vi "Lockin.Engine.vi"(8 "error in (no error)":errorcluster, 11 "Instrument.DAQ":refnum<class "Instrument.DAQ.lvclass">) -> (0 "error out":errorcluster, 1 "Downsampled Waveforms":T1, 2 "Results (X,Y,R,Theta,Mean)":T2 {"Results (Dictionary)"."value" format="%#_6p"}, 3 "Instrument.DAQ out":refnum<class "Instrument.DAQ.lvclass">, 5 "Continue DSP?":bool)   [LabVIEW 2019, in "Instrument.Lockin.lvlib" / "Instrument.DAQ.lvclass"]
uses:
  Instrument.DAQ.lvclass
  Typedefs/Results--Cluster.ctl
  Instrument.DAQ.lvclass/Instrument.DAQ.ctl
  DSP/DSP.lvclass
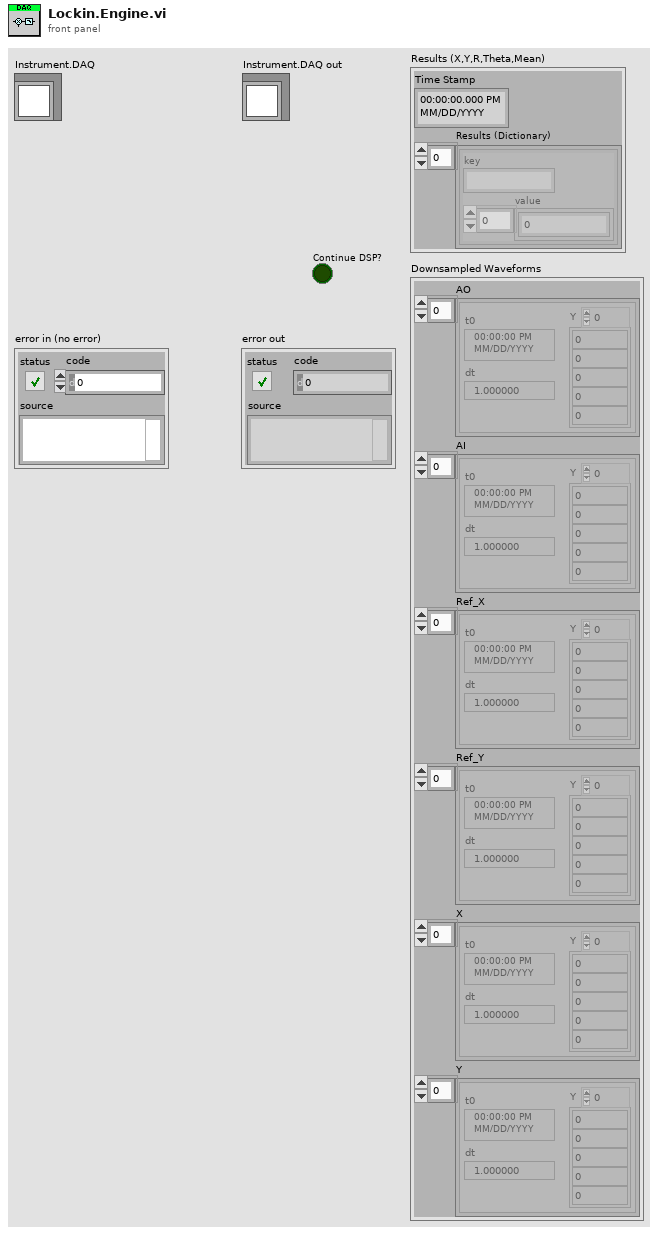
[diagram p1: front panel]
types:
  T1 = cluster{"AO":waveform(dbl)[], "AI":waveform(dbl)[], "Ref_X":waveform(dbl)[], "Ref_Y":waveform(dbl)[], "X":waveform(dbl)[], "Y":waveform(dbl)[]}
  T2 = typedef "Instrument.Lockin.lvlib/Instrument.DAQ.lvclass/Results--Cluster.ctl" = cluster{"Time Stamp":timestamp, "Results (Dictionary)":cluster{"key":string, "value":dbl[]}[]}
  T3 = typedef "Instrument.Lockin.lvlib/Instrument.DAQ.lvclass/PublicEvents--DAQ.getWaveforms.ctl" = cluster{"AO":waveform(dbl)[], "AI":waveform(dbl)[], "REF_X":waveform(dbl)[], "REF_Y":waveform(dbl)[], "X":waveform(dbl)[], "Y":waveform(dbl)[]}
  T4 = typedef "Instrument.Lockin.lvlib/Instrument.DAQ.lvclass/AI.Channel--Cluster--Array.ctl" = T5[]
  T5 = typedef "Instrument.Lockin.lvlib/Instrument.DAQ.lvclass/AI.Channel--Cluster.ctl" = cluster{"Enable?":bool, "Channel":i32, "References":u16[], "reference index":i32}
  T6 = typedef "Instrument.Lockin.lvlib/Instrument.DAQ.lvclass/REF.Channel--Cluster--Array.ctl" = T7[]
  T7 = typedef "Instrument.Lockin.lvlib/Instrument.DAQ.lvclass/REF.Channel--Cluster.ctl" = cluster{"Enable?":bool, "Channel":i32, "Frequency":dbl, "Phase":dbl, "TC":dbl, "Roll-Off":i32}
  T8 = typedef "Instrument.Lockin.lvlib/Instrument.DAQ.lvclass/DAQ.Sampling--Cluster.ctl" = cluster{"Sampling":T9, "Fs_Out":dbl}
  T9 = typedef "Instrument.Lockin.lvlib/Instrument.DAQ.lvclass/DAQ.Sampling.Sampling--Cluster.ctl" = cluster{"Fs":dbl, "#s":i32}
  T10 = typedef "DSP.lvclass/Results--Cluster.ctl" = cluster{"Time Stamp":timestamp, "Results (Dictionary)":T11[]}
  T11 = typedef "DSP.lvclass/Results Dictionary--Cluster.ctl" = cluster{"key":string, "value":dbl[]}
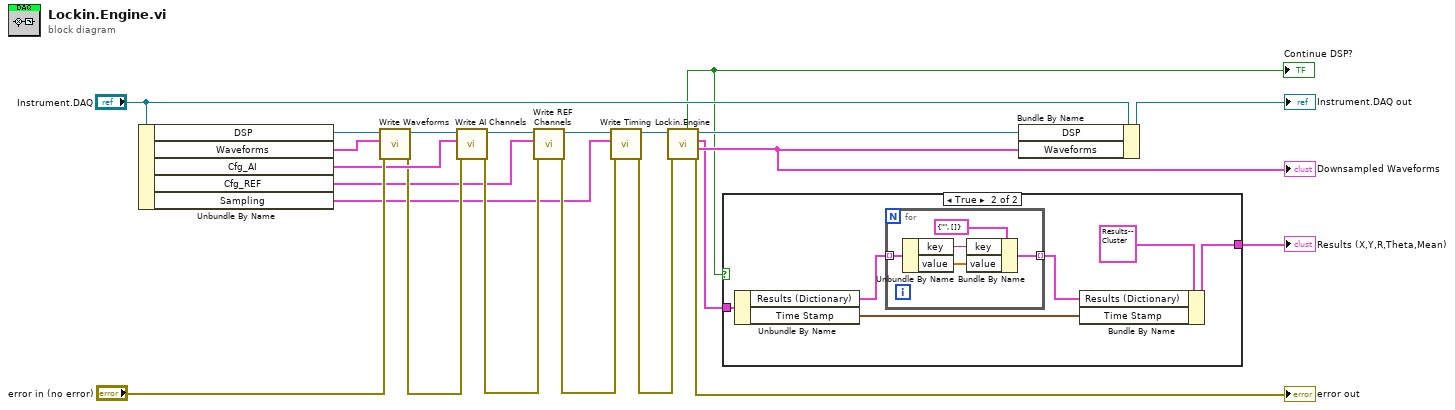
[diagram p0: block diagram]
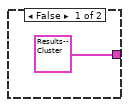
[diagram p2: hidden frame]
diagram:
  n1 = Unbundle By Name("Instrument.DAQ") -> ("DSP"=w19:refnum<class "DSP.lvclass">, "Waveforms"=w17:T3, "Cfg_AI"=w16:T4, "Cfg_REF"=w7:T6, "Sampling"=w6:T8)
  n2 = call "Write Waveforms.vi"("error in (no error)"="error in (no error)", "Waveforms"=w17, "DSP in"=w19) -> ("error out"=w15:errorcluster, "DSP out"=w13:refnum<class "DSP.lvclass">)  [unwired: 7 in]
  n3 = call "Write AI Channels.vi"("error in (no error)"=w15, "AI Channels"=w16, "DSP in"=w13) -> ("error out"=w11:errorcluster, "DSP out"=w12:refnum<class "DSP.lvclass">)  [unwired: 7 in]
  n4 = call "Write REF Channels.vi"("error in (no error)"=w11, "REF Channels"=w7, "DSP in"=w12) -> ("error out"=w9:errorcluster, "DSP out"=w10:refnum<class "DSP.lvclass">)  [unwired: 7 in]
  n5 = call "Write Timing.vi"("error in (no error)"=w9, "Timing"=w6, "DSP in"=w10) -> ("error out"=w14:errorcluster, "DSP out"=w8:refnum<class "DSP.lvclass">)  [unwired: 7 in]
  n6 = call "Lockin.Engine.vi"("error in (no error)"=w14, "DSP in"=w8) -> ("error out"=→"error out":errorcluster, "Downsampled Waveforms"=w4:T1, "Results"=w1:T10, "DSP out"=w21:refnum<class "DSP.lvclass">, "Continue DSP?"=w2:bool)  [unwired: 5 in]
  "Downsampled Waveforms" <- w4
  "Continue DSP?" <- w2
  n7 = case shown="True" w2 {
    tunnel: [T2 {"Time Stamp"=timestamp(0 s since 1904-01-01), "Results (Dictionary)"=[]} ("<Results> (X,Y,R,Theta,Mean)") w27] -> w5
    tunnel: w1 -> [_ w24]
    frame False {
    }
    frame True {
      n8 = Unbundle By Name(w24) -> ("Results (Dictionary)"=w25:T11[], "Time Stamp"=w29:timestamp)
      n9 = for {
        tunnel: w25 -> [w34] mode=indexing
        tunnel: [w32] -> w26 mode=indexing
        n10 = Unbundle By Name(w34) -> ("key"=w31:string, "value"=w33:dbl[])
        n11 = Bundle By Name(cluster=cluster{"key":string, "value":dbl[]} {"key"="", "value"=[]} ("element"), "key"=w31, "value"=w33) -> (w32:cluster{"key":string, "value":dbl[]})
      }
      n12 = Bundle By Name(cluster=T2 {"Time Stamp"=timestamp(0 s since 1904-01-01), "Results (Dictionary)"=[]} ("<Results> (X,Y,R,Theta,Mean)"), "Results (Dictionary)"=w26, "Time Stamp"=w29) -> (w27:T2)
    }
  }
  "Results (X,Y,R,Theta,Mean)" <- w5
  n13 = Bundle By Name(cluster="Instrument.DAQ", "DSP"=w21, "Waveforms"=w4) -> (→"Instrument.DAQ out":refnum<class "Instrument.DAQ.lvclass">)
